vi "List columns.vi"(8 "error in (no error)":errorcluster, 9 "显示关键参数":bool, 10 "table":string, 11 "database":string="database1.mdb") -> (0 "error out":errorcluster, 3 "columns":string[](array[string]))   [LabVIEW 2016, in "数据查询.lvlib"]
uses:
  <vilib>/addons/database/Connection.llb/DB Tools Open Connec (String).vi
  <userlib>/_LVST/sqlite_api/Core/Tables/SQLite_List Columns.vi
  <userlib>/_OpenG.lib/array/array.llb/Filter 1D Array (String)__ogtk.vi
  <vilib>/addons/database/NI_Database_API.lvlib
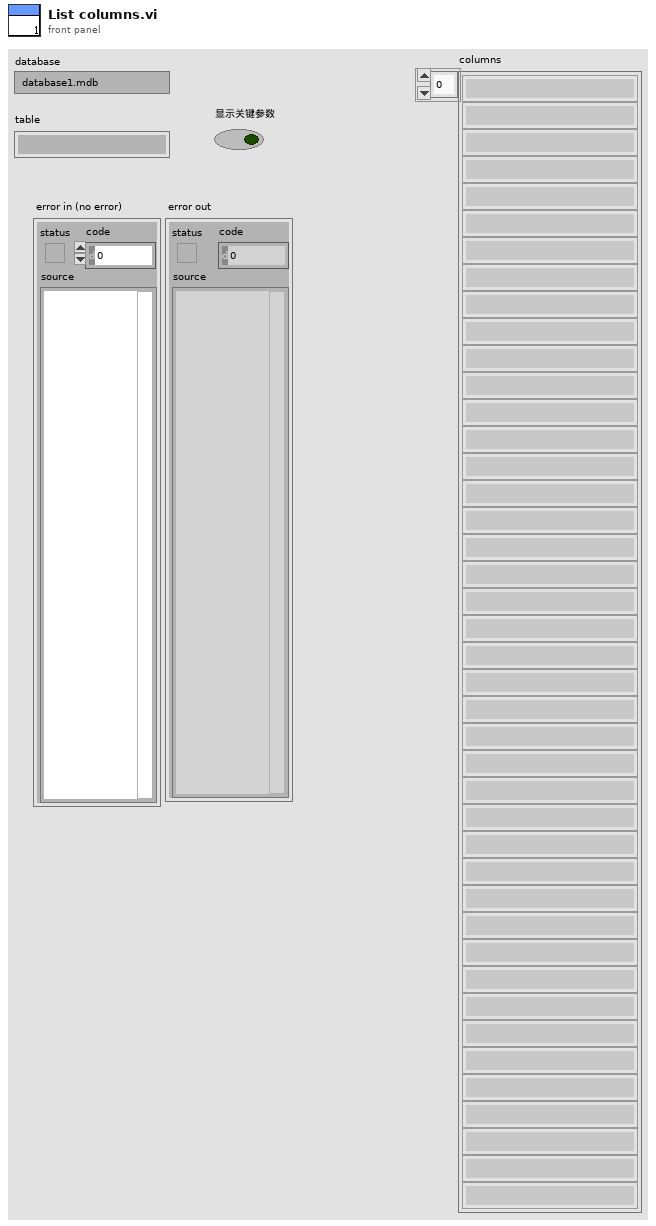
[diagram p1: front panel]
types:
  T1 = typedef "数据库类型.ctl" = enum16{"Access", "SQLite"}
  T2 = typedef "NI_Database_API.lvlib/Conn ObjectReference.ctl" = refnum<k1>
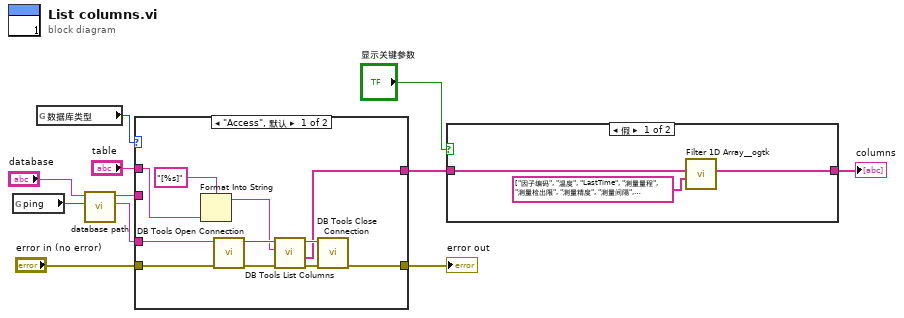
[diagram p0: block diagram]
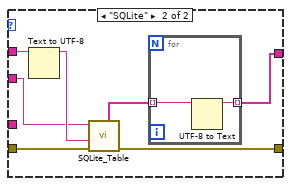
[diagram p3: hidden frame]
diagram:
  n1 = global read "全局变量.vi" "ping"() -> (w6:bool)
  n2 = global read "外部调用接口全局变量.vi" "数据库类型"() -> (w1:T1)
  n3 = call "database path.vi"("ping"=w6, "database"="database") -> ("Connection information"=w2:string, "Path out"=w7:string)  [unwired: 8 in]
  n4 = case shown="\"Access\", 默认" w1 {
    tunnel: "table" -> [w13 w25]
    tunnel: "error in (no error)" -> [w18 w28]
    tunnel: [w17 w29] -> w9
    tunnel: [w16 w26] -> w4
    tunnel: w7 -> [_ w23]
    tunnel: w2 -> [w15 _]
    frame "Access", Default {
      n5 = Format Into String(format string="[%s]" ("格式字符串"), w13) -> (resulting string=w14:string)  [unwired: 2 in, 1 out]
      n6 = call-poly <vilib>:"DB Tools Open Connection.vi"("error in (no error)"=w18, "connection information"=w15) -> ("error out"=w20:errorcluster, "connection reference"=w22:T2)  [unwired: 6 in]
      n7 = call <vilib>:"DB Tools List Columns.vi"("error in (no error)"=w20, "table"=w14, "connection reference"=w22) -> ("error out"=w19:errorcluster, "columns"=w16:string[], "connection reference out"=w21:T2)  [unwired: 1 in, 1 out]
      n8 = call <vilib>:"DB Tools Close Connection.vi"("error in (no error)"=w19, "connection reference"=w21) -> ("error out"=w17:errorcluster)  [unwired: 5 in]
    }
    frame "SQLite" {
      n9 = Text to UTF-8(11:w25) -> (3:w24:string)  [unwired: 2 in, 1 out]
      n10 = call-poly <userlib>:"SQLite_Table.vi"("DB Path"=w23, "Table Name"=w24, "error in (no error)"=w28) -> ("Columns"=w27:string[], "error out"=w29:errorcluster)  [unwired: 4 in, 2 out]
      n11 = for {
        tunnel: w27 -> [w31] mode=indexing
        tunnel: [w30] -> w26 mode=indexing
        n12 = UTF-8 to Text(11:w31) -> (3:w30:string)  [unwired: 2 in, 1 out]
      }
    }
  }
  "error out" <- w9
  n13 = case shown="假" "显示关键参数" {
    tunnel: w4 -> [w34 w35]
    tunnel: [w32 w35] -> w3
    frame False {
      n14 = call-poly <userlib>:"Filter 1D Array__ogtk.vi"("items to filter"=string[] ["因子编码", "温度", "LastTime", "测量量程", "测量检出限", "测量精度", "测量间隔", "消解温度", "消解时长", "三项式系数", "二次多项式系数", "曲线斜率", "曲线截距", "线性相关系数", "空白校准时间", "标样校准时间", "测量信号值", "稀释倍数", "空白标定系数", "量程系数", "X1"] ("columns"), "array"=w34) -> ("filtered array"=w32:string[])  [unwired: 4 in, 1 out]
    }
    frame True {
    }
  }
  "columns" <- w3
